vi "Connect in POLL Mode.vi"(8 "error in":errorcluster, 11 "Vaisala in":refnum<class "Vaisala.lvclass">) -> (0 "error out":errorcluster, 3 "Vaisala out":refnum<class "Vaisala.lvclass">)   [LabVIEW 2014, in "Vaisala Library.lvlib" / "Vaisala.lvclass"]
uses:
  Vaisala.lvclass
  Vaisala.lvclass/Vaisala.ctl
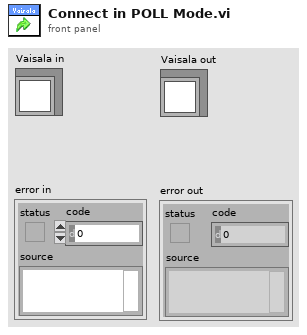
[diagram p1: front panel]
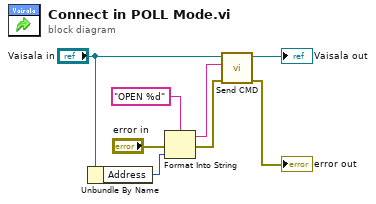
[diagram p0: block diagram]
diagram:
  n1 = Unbundle By Name("Vaisala in") -> ("Address"=w8:u8)
  n2 = Format Into String(format string="OPEN %d", error in="error in", w8) -> (resulting string=w5:string, error out=w4:errorcluster)  [unwired: 1 in]
  n3 = call "Send CMD.vi"("error in"=w4, "CMD In"=w5, "Vaisala in"="Vaisala in") -> ("error out"=→"error out":errorcluster, "Vaisala out"=→"Vaisala out":refnum<class "Vaisala.lvclass">)  [unwired: 7 in]
